vi "read_write_arduino.vi"(0 "VISA in":refnum<visa-resource-name>, 5 "Pin Num":u8=2 min=2 max=12, 7 "Read (0, default)/Write (1)":bool, 9 "State":bool, 11 "error in":errorcluster) -> (4 "VISA out":refnum<visa-resource-name>, 8 "State":bool, 10 "Comms Reset":bool, 15 "error out":errorcluster)   [LabVIEW 2018]
uses:
  CAEN globals.vi
panel:
  in  "Long Read":bool
  out "Bytes at Port":u32
  out "read buffer":string
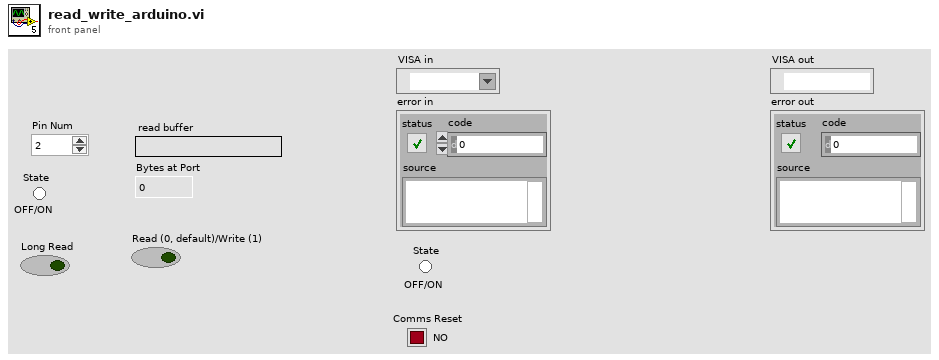
[diagram p1: front panel]
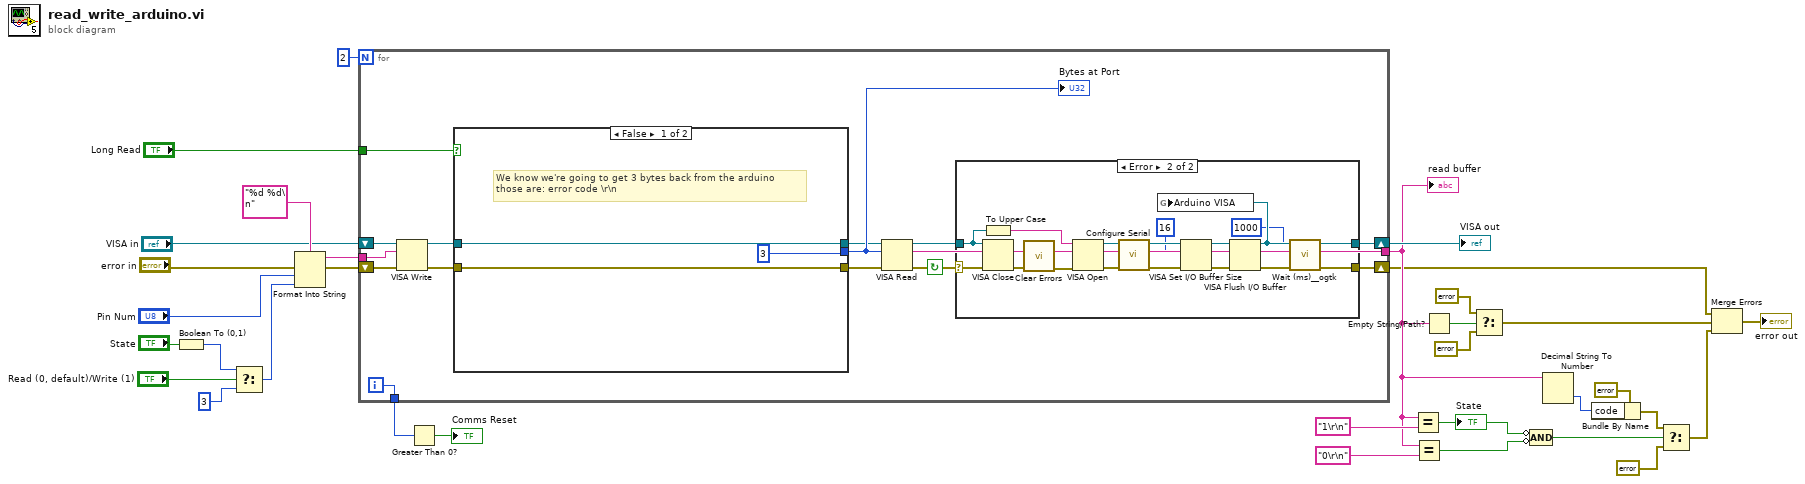
[diagram p0: block diagram]
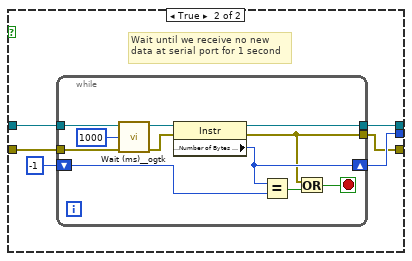
[diagram p3: hidden frame]
diagram:
  n1 = Boolean To (0,1)(Boolean="State") -> (0, 1=w4:i16)
  n2 = Select(t=w4, s="Read (0, default)/Write (1)", f=i16 3 ("t")) -> (s? t:f=w24:i16)
  n3 = Format Into String(format string="%d %d\n", error in="error in", "Pin Num", w24) -> (resulting string=w32:string, error out=w33:errorcluster)  [unwired: 1 in]
  n4 = for {
    N: 2 -> [_]
    tunnel: w32 -> [w47]
    tunnel: "Long Read" -> [w43]
    tunnel: [w39] -> w12
    shift-right: [w38] -> w9
    shift-left: w33 -> [w48]
    shift-right: [w37] -> w28
    shift-left: "VISA in" -> [w46]
    tunnel: [w34] -> w2
    i -> [w34]
    stop <- w35 continue-if-true
    n5 = VISA Write(VISA resource name=w46, write buffer=w47, error in (no error)=w48) -> (VISA resource name out=w44:refnum<visa-resource-name>, error out=w45:errorcluster)  [unwired: 1 out]
    n6 = case shown="False" w43 {
      tunnel: w45 -> [w68 w75]
      tunnel: w44 -> [w67 w74]
      tunnel: [u32 3 ("Bytes at Port") w72] -> w42
      tunnel: [w67 w71] -> w41
      tunnel: [w68 w70] -> w40
      frame False {
        # "We know we're going to get 3 bytes back from the arduino\nthose are: error code \\r\\n"
      }
      frame True {
        # "Wait until we receive no new \ndata at serial port for 1 second"
        n7 = while {
          tunnel: w74 -> [w85]
          tunnel: w75 -> [w82]
          shift-right: [w80] -> w72
          shift-left: -1 ("timeout (10sec)") -> [w81]
          tunnel: [w79] -> w71
          tunnel: [w76] -> w70
          stop <- w78 stop-if-true
          n8 = call <userlib>:"Wait (ms)__ogtk.vi"("error in (no error)"=w82, "milliseconds to wait"=u32 1000) -> ("error out"=w83:errorcluster)  [unwired: 8 in, 1 out]
          n9 = property class="Instr"(reference=w85, error in=w83) -> (reference out=w79:refnum<visa-resource-name>, error out=w76:errorcluster, "Serial Settings:Number of Bytes at Serial Port"=w80:u32)
          n10 = Equal?(x=w80, y=w81) -> (x = y?=w77:bool)
          n11 = Or(x=w76, y=w77) -> (x .or. y?=w78:bool)
        }
      }
    }
    "Bytes at Port" <- w42
    n12 = VISA Read(VISA resource name=w41, byte count=w42, error in (no error)=w40) -> (VISA resource name out=w36:refnum<visa-resource-name>, read buffer=w39:string, error out=w35:errorcluster)  [unwired: 1 out]
    n13 = case shown="Error" w35 {
      selector: w35 -> [w50 w60]
      tunnel: [w50 w54] -> w38
      tunnel: [w49 w61] -> w37
      tunnel: w36 -> [w49 w57]
      frame No Error {
      }
      frame Error {
        n14 = To Upper Case(1:w57) -> (0:w56:string)
        n15 = VISA Close(VISA resource name=w57, error in (no error)=w60) -> (error out=w52:errorcluster)
        n16 = call <vilib>:"Clear Errors.vi"("error in (no error)"=w52) -> ("error out"=w51:errorcluster)  [unwired: 5 in, 1 out]
        n17 = VISA Open(error in (no error)=w51, VISA resource name=w56) -> (VISA resource name=w58:refnum<visa-resource-name>, error out=w59:errorcluster)  [unwired: 3 in]
        n18 = call "Configure Serial.vi"("error in"=w59, "Resource Name"=w58) -> ("error out"=w62:errorcluster, "VISA out"=w66:refnum<visa-resource-name>)  [unwired: 8 in]
        n19 = VISA Set I/O Buffer Size(VISA resource name=w66, mask (16)=u16 16 ("I/O Receive\nBuffer mask"), error in (no error)=w62) -> (VISA resource name out=w65:refnum<visa-resource-name>, error out=w63:errorcluster)  [unwired: 1 in]
        n20 = VISA Flush I/O Buffer(VISA resource name=w65, error in (no error)=w63) -> (VISA resource name out=w61:refnum<visa-resource-name>, error out=w55:errorcluster)  [unwired: 1 in]
        n21 = global write "CAEN globals.vi" "Arduino VISA"(w61) -> ()
        n22 = call <userlib>:"Wait (ms)__ogtk.vi"("error in (no error)"=w55, "milliseconds to wait"=u32 1000 ("I/O Receive\nBuffer mask")) -> ("error out"=w54:errorcluster)  [unwired: 8 in, 1 out]
      }
    }
  }
  "read buffer" <- w12
  "VISA out" <- w28
  n23 = Greater Than 0?(x=w2) -> (x > 0?=→"Comms Reset":bool)
  n24 = Equal?(x=w12, y="1\r\n" ("read buffer")) -> (x = y?=w16:bool)
  "State" <- w16
  n25 = Equal?(x=w12, y="0\r\n" ("read buffer")) -> (x = y?=w15:bool)
  n26 = Empty String/Path?(string/path=w12) -> (empty?=w22:bool)
  n27 = Select(t=errorcluster {"status"=TRUE, "code"=0, "source"="No response from arduino!"} ("error out"), s=w22, f=errorcluster {"status"=FALSE, "code"=0, "source"=""} ("error out")) -> (s? t:f=w19:errorcluster)
  n28 = Compound Arithmetic op=AND(invert w16, invert w15) -> (w14:bool)
  n29 = Decimal String To Number(string=w12) -> (number=w11:i32)  [unwired: 2 in, 1 out]
  n30 = Bundle By Name(cluster=errorcluster {"status"=TRUE, "code"=0, "source"="Error code from arduino!"} ("error out"), "code"=w11) -> (w8:errorcluster)
  n31 = Select(t=w8, s=w14, f=errorcluster {"status"=FALSE, "code"=0, "source"=""} ("error out")) -> (s? t:f=w7:errorcluster)
  n32 = Merge Errors(w9, w19, w7) -> (→"error out":errorcluster)
